vi "[Teste]CaseSelect.vi"() -> ()   [LabVIEW 2014]
panel:
  out "String":string
  in  "Voltagem":dbl
  in  "Condutividade":dbl
  out "Adssorção":bool
  in  "Liga/Desliga":bool
  out "Dessorção":bool
  out "Single-Pass":bool
  out "Batch":bool
  in  "BATCH / SINGLE PASS":bool
  in  "?":T1(tab)
  in  "CONDUTIVIDADE \nMÁXIMA NA DESSORÇÃO P":dbl
  in  "TEMPO DE DESSOR敲O P":dbl
  in  "CONDUTIVIDADE \nMÍNIMA NA ADSORÇÃO P":dbl
  in  "TEMPO DE ADSOR敲O P":dbl
  in  "POTENCIAL DE CORTE\nNA DESSOR敲O (V) G":dbl
  in  "POTENCIAL DE CORTE\nNA ADSOR敲O (V) G":dbl
  in  "CONDUTIVIDADE \nMÁXIMA NA DESSORÇÃO G":dbl
  in  "TEMPO DE DESSOR敲O G":dbl
  in  "CONDUTIVIDADE \nMÍNIMA NA ADSORÇÃO G":dbl
  in  "TEMPO DE ADSOR敲O G":dbl
  in  "Selecionar parämetro G":enum32{"Tempo", "Condutividade", "Potencial"}(tab)
  in  "TEMPO DE DESSOR敲O G2":dbl
  in  "TEMPO DE ADSOR敲O G2":dbl
  in  "CONDUTIVIDADE \nMÁXIMA NA DESSORÇÃO G2":dbl
  in  "CONDUTIVIDADE \nMÍNIMA NA ADSORÇÃO G2":dbl
  in  "POTENCIAL DE CORTE\nNA DESSOR敲O G2":dbl
  in  "POTENCIAL DE CORTE\nNA ADSOR敲O G2":dbl
  # "s"
  # "s"
  # "us/cm"
  # "s"
  # "us/cm"
  # "s"
  # "s"
  # "us/cm"
  # "us/cm"
  # "VV"
  # "V"
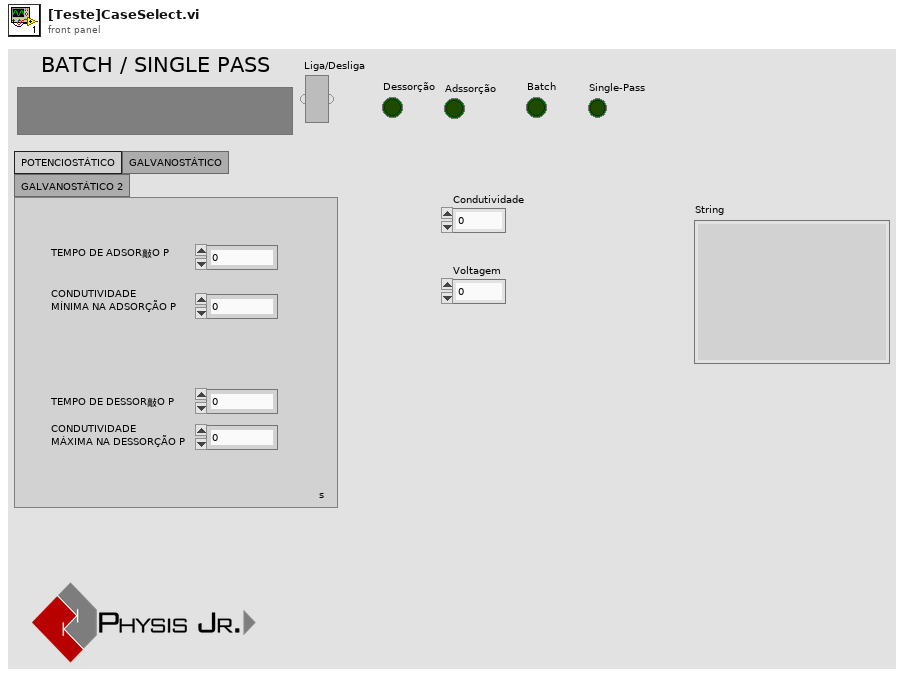
[diagram p1: front panel]
types:
  T1 = enum32{"POTENCIOSTÁTICO", "GALVANOSTÁTICO", "GALVANOSTÁTICO 2"}
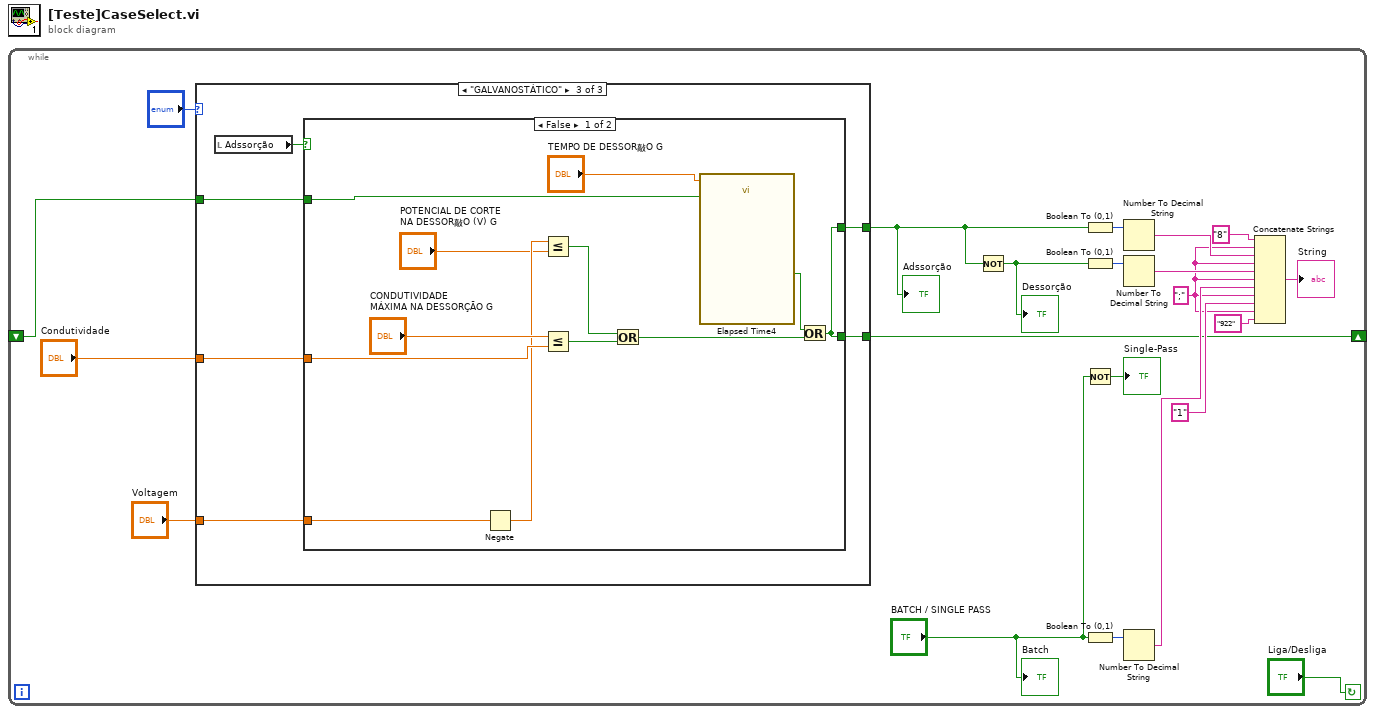
[diagram p0: block diagram]
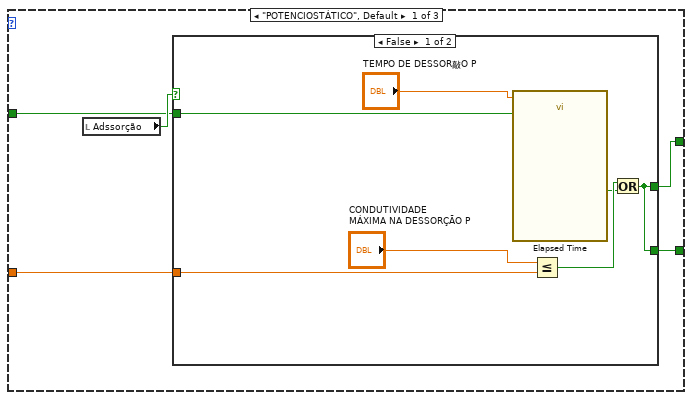
[diagram p2: hidden frame]
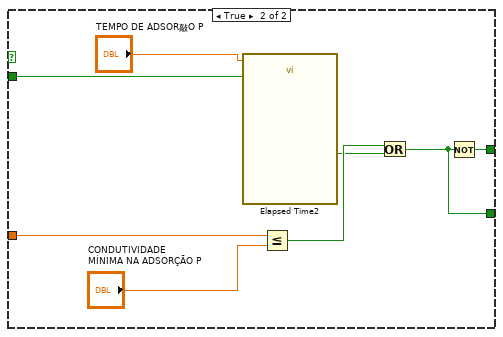
[diagram p3: hidden frame]
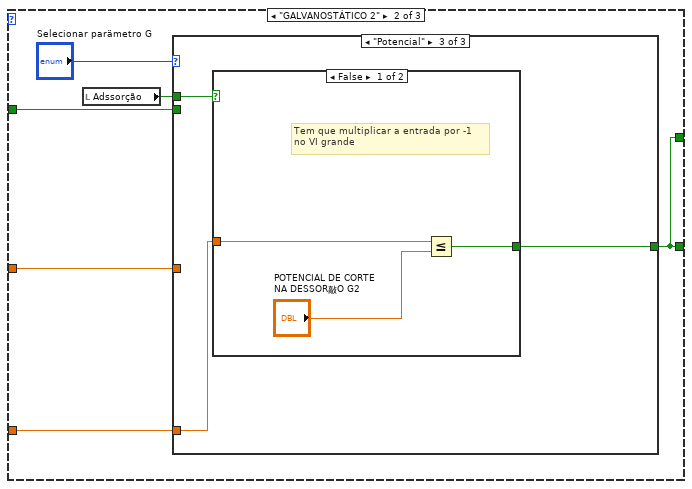
[diagram p4: hidden frame]
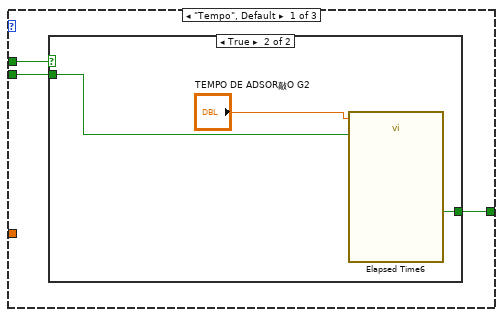
[diagram p5: hidden frame]
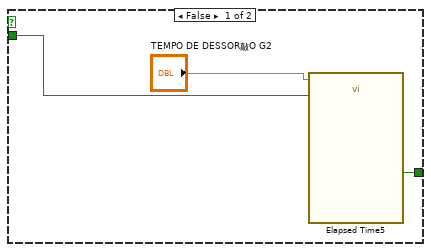
[diagram p6: hidden frame]
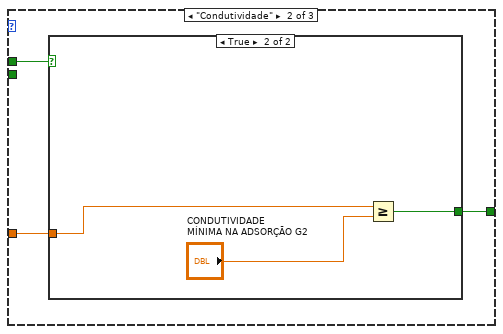
[diagram p7: hidden frame]
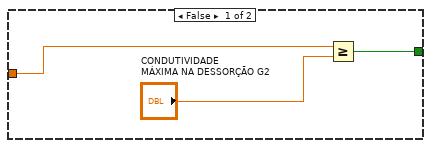
[diagram p8: hidden frame]
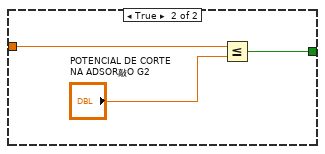
[diagram p9: hidden frame]
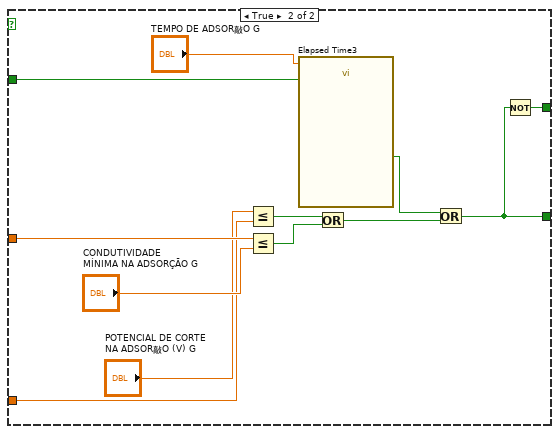
[diagram p10: hidden frame]
diagram:
  n1 = while {
    shift-right: [w2] -> _
    shift-left: _ -> [w1]
    stop <- "Liga/Desliga" continue-if-true
    w6 = ";"
    n2 = case shown="\"GALVANOSTÁTICO\"" "?" {
      tunnel: "Condutividade" -> [w25 w43 w79]
      tunnel: "Voltagem" -> [_ w42 w78]
      tunnel: [w24 w44 w77] -> w15
      tunnel: [w23 w44 w76] -> w2
      tunnel: w1 -> [w22 w45 w75]
      frame "POTENCIOSTÁTICO", Default {
        n3 = local read "Adssorção"() -> (w26:bool)
        n4 = case shown="False" w26 {
          tunnel: w25 -> [w31 w40]
          tunnel: [w27 w36] -> w24
          tunnel: [w27 w34] -> w23
          tunnel: w22 -> [w28 w35]
          frame False {
            n5 = call "Elapsed Time"("Time Target (s)"="TEMPO DE DESSOR敲O P", "Reset"=w28) -> ("Time has Elapsed"=w29:bool)  [unwired: 10 in, 7 out]
            n6 = Less Or Equal?(x="CONDUTIVIDADE \nMÁXIMA NA DESSORÇÃO P", y=w31) -> (x <= y?=w30:bool)
            n7 = Or(x=w30, y=w29) -> (x .or. y?=w27:bool)
          }
          frame True {
            n8 = call "Elapsed Time2"("Time Target (s)"="TEMPO DE ADSOR敲O P", "Reset"=w35) -> ("Time has Elapsed"=w37:bool)  [unwired: 10 in, 7 out]
            n9 = Less Or Equal?(x=w40, y="CONDUTIVIDADE \nMÍNIMA NA ADSORÇÃO P") -> (x <= y?=w38:bool)
            n10 = Or(x=w38, y=w37) -> (x .or. y?=w34:bool)
            n11 = Not(x=w34) -> (.not. x?=w36:bool)
          }
        }
      }
      frame "GALVANOSTÁTICO 2" {
        n12 = local read "Adssorção"() -> (w46:bool)
        n13 = case shown="\"Potencial\"" "Selecionar parämetro G" {
          tunnel: w46 -> [w50 w59 w68]
          tunnel: w45 -> [w49 _ _]
          tunnel: [w48 w57 w67] -> w44
          tunnel: w43 -> [_ w58 _]
          tunnel: w42 -> [_ _ w66]
          frame "Tempo", Default {
            n14 = case shown="True" w50 {
              tunnel: w49 -> [w52 w54]
              tunnel: [w51 w55] -> w48
              frame False {
                n15 = call "Elapsed Time5"("Time Target (s)"="TEMPO DE DESSOR敲O G2", "Reset"=w52) -> ("Time has Elapsed"=w51:bool)  [unwired: 10 in, 7 out]
              }
              frame True {
                n16 = call "Elapsed Time6"("Time Target (s)"="TEMPO DE ADSOR敲O G2", "Reset"=w54) -> ("Time has Elapsed"=w55:bool)  [unwired: 10 in, 7 out]
              }
            }
          }
          frame "Condutividade" {
            n17 = case shown="True" w59 {
              tunnel: w58 -> [w62 w65]
              tunnel: [w60 w63] -> w57
              frame False {
                n18 = Greater Or Equal?(x=w62, y="CONDUTIVIDADE \nMÁXIMA NA DESSORÇÃO G2") -> (x >= y?=w60:bool)
              }
              frame True {
                n19 = Greater Or Equal?(x=w65, y="CONDUTIVIDADE \nMÍNIMA NA ADSORÇÃO G2") -> (x >= y?=w63:bool)
              }
            }
          }
          frame "Potencial" {
            n20 = case shown="False" w68 {
              tunnel: [w70 w73] -> w67
              tunnel: w66 -> [w69 w72]
              frame False {
                # "Tem que multiplicar a entrada por -1\nno VI grande"
                n21 = Less Or Equal?(x=w69, y="POTENCIAL DE CORTE\nNA DESSOR敲O G2") -> (x <= y?=w70:bool)
              }
              frame True {
                n22 = Less Or Equal?(x=w72, y="POTENCIAL DE CORTE\nNA ADSOR敲O G2") -> (x <= y?=w73:bool)
              }
            }
          }
        }
      }
      frame "GALVANOSTÁTICO" {
        n23 = local read "Adssorção"() -> (w80:bool)
        n24 = case shown="False" w80 {
          tunnel: w79 -> [w90 w98]
          tunnel: w78 -> [w83 w94]
          tunnel: [w85 w103] -> w77
          tunnel: [w85 w100] -> w76
          tunnel: w75 -> [w84 w99]
          frame False {
            n25 = Negate(x=w83) -> (-x=w82:dbl)
            n26 = Less Or Equal?(x=w82, y="POTENCIAL DE CORTE\nNA DESSOR敲O (V) G") -> (x <= y?=w89:bool)
            n27 = Less Or Equal?(x="CONDUTIVIDADE \nMÁXIMA NA DESSORÇÃO G", y=w90) -> (x <= y?=w88:bool)
            n28 = Or(x=w89, y=w88) -> (x .or. y?=w87:bool)
            n29 = call "Elapsed Time4"("Time Target (s)"="TEMPO DE DESSOR敲O G", "Reset"=w84) -> ("Time has Elapsed"=w86:bool)  [unwired: 10 in, 7 out]
            n30 = Or(x=w86, y=w87) -> (x .or. y?=w85:bool)
          }
          frame True {
            n31 = Less Or Equal?(x="POTENCIAL DE CORTE\nNA ADSOR敲O (V) G", y=w94) -> (x <= y?=w93:bool)
            n32 = Less Or Equal?(x=w98, y="CONDUTIVIDADE \nMÍNIMA NA ADSORÇÃO G") -> (x <= y?=w96:bool)
            n33 = call "Elapsed Time3"("Time Target (s)"="TEMPO DE ADSOR敲O G", "Reset"=w99) -> ("Time has Elapsed"=w101:bool)  [unwired: 10 in, 7 out]
            n34 = Or(x=w93, y=w96) -> (x .or. y?=w102:bool)
            n35 = Or(x=w101, y=w102) -> (x .or. y?=w100:bool)
            n36 = Not(x=w100) -> (.not. x?=w103:bool)
          }
        }
      }
    }
    "Adssorção" <- w15
    n37 = Not(x=w15) -> (.not. x?=w12:bool)
    "Dessorção" <- w12
    n38 = Boolean To (0,1)(Boolean=w15) -> (0, 1=w16:i16)
    n39 = Boolean To (0,1)(Boolean=w12) -> (0, 1=w13:i16)
    n40 = Not(x="BATCH / SINGLE PASS") -> (.not. x?=→"Single-Pass":bool)
    n41 = Boolean To (0,1)(Boolean="BATCH / SINGLE PASS") -> (0, 1=w10:i16)
    n42 = Number To Decimal String(number=w16) -> (decimal integer string=w14:string)  [unwired: 1 in]
    n43 = Number To Decimal String(number=w13) -> (decimal integer string=w11:string)  [unwired: 1 in]
    n44 = Number To Decimal String(number=w10) -> (decimal integer string=w8:string)  [unwired: 1 in]
    n45 = Concatenate Strings("8", w6, w14, w6, w11, w6, w8, w6, "1", w6, "922") -> (→"String":string)
    "Batch" <- "BATCH / SINGLE PASS"
  }
